vi "ParsePacket.vi"(0 "data out":string) -> (1 "Node ID":u8, 2 "Source Type":u8, 3 "CO2":u16, 4 "Light":u16, 5 "Humidity":u16, 6 "Temperature":u16)   [LabVIEW 2011]
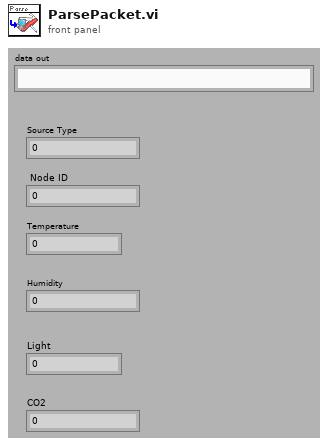
[diagram p1: front panel]
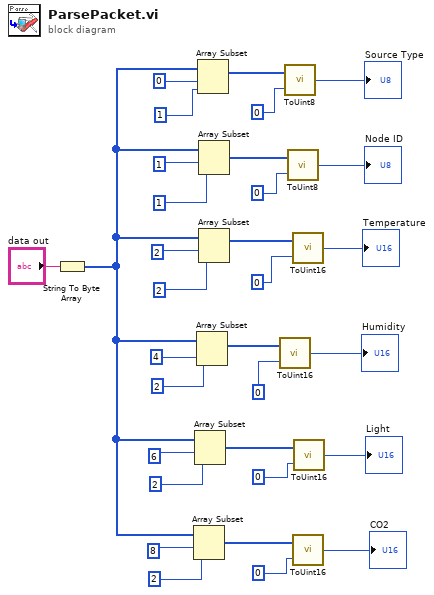
[diagram p0: block diagram]
diagram:
  n1 = String To Byte Array(string="data out") -> (unsigned byte array=w10:u8[])
  n2 = Array Subset(array=w10, index=8 ("x"), length=2 ("x")) -> (w14:u8[])
  n3 = Array Subset(array=w10, index=6 ("x"), length=2 ("x")) -> (w23:u8[])
  n4 = Array Subset(array=w10, index=4 ("x"), length=2 ("x")) -> (w28:u8[])
  n5 = Array Subset(array=w10, index=0, length=1) -> (w8:u8[])
  n6 = Array Subset(array=w10, index=1 ("length"), length=1) -> (w7:u8[])
  n7 = Array Subset(array=w10, index=2 ("x"), length=2 ("x")) -> (w15:u8[])
  n8 = call "ToUint16.vi"("index"=0 ("x"), "array"=w28) -> ("sp float"=→"Humidity":u16)
  n9 = call "ToUint8.vi"("index"=0, "array"=w8) -> ("sp float"=→"Source Type":u8)
  n10 = call "ToUint8.vi"("index"=0, "array"=w7) -> ("sp float"=→"Node ID":u8)
  n11 = call "ToUint16.vi"("index"=0, "array"=w15) -> ("sp float"=→"Temperature":u16)
  n12 = call "ToUint16.vi"("index"=0, "array"=w14) -> ("sp float"=→"CO2":u16)
  n13 = call "ToUint16.vi"("index"=0, "array"=w23) -> ("sp float"=→"Light":u16)
